vi "TREE_output the selected item.vi"(8 "error in":errorcluster, 10 "only if double click (F)":bool, 11 "Tree In":refnum<vi>) -> (0 "error out":errorcluster, 1 "selected item":string, 2 "selectrd item (path)":path, 3 "Tree Out":refnum<vi>, 4 "directory file names":string[](array[string]))   [LabVIEW 2011]
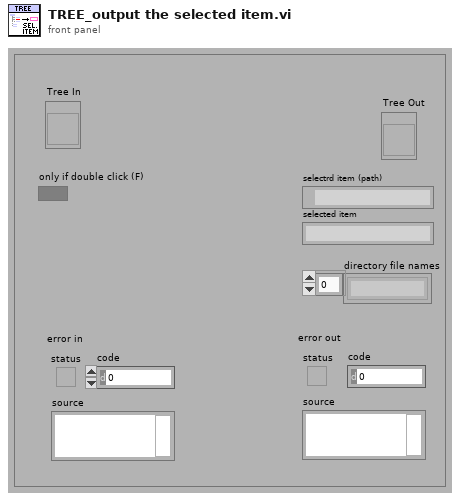
[diagram p1: front panel]
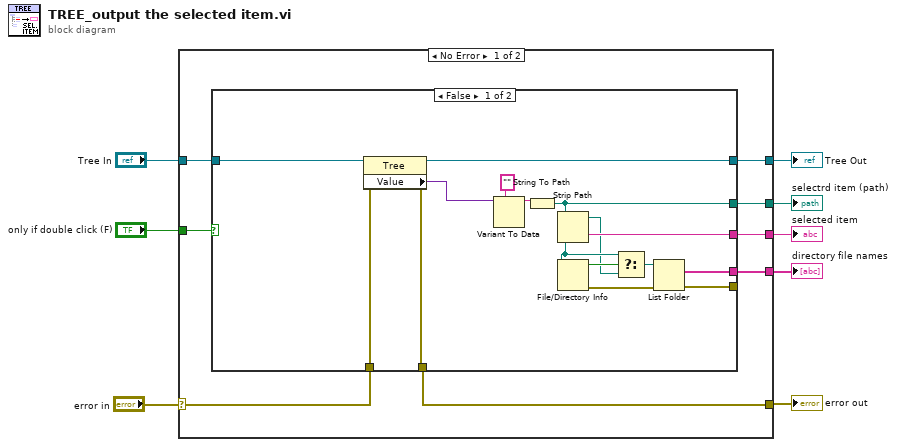
[diagram p0: block diagram]
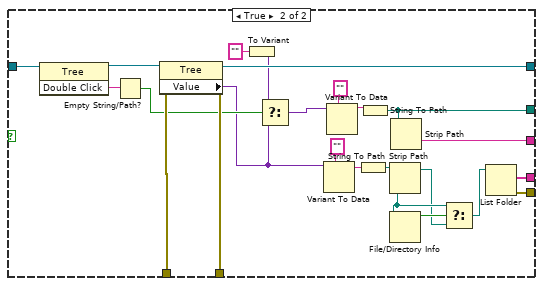
[diagram p2: hidden frame]
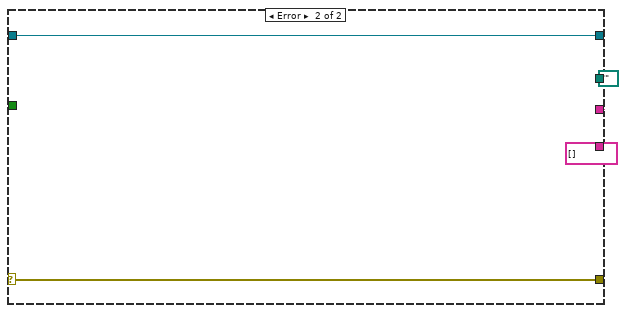
[diagram p3: hidden frame]
diagram:
  n1 = case shown="No Error" "error in" {
    selector: "error in" -> [w15 w58]
    tunnel: "Tree In" -> [w10 w57]
    tunnel: [w10 w57] -> w7
    tunnel: [w9 w58] -> w6
    tunnel: [w14 path ""] -> w4
    tunnel: [w13 "" ("name")] -> w3
    tunnel: "only if double click (F)" -> [w11 _]
    tunnel: [w12 string[] [] ("directory names")] -> w1
    frame No Error {
      n2 = case shown="False" w11 {
        tunnel: [w24 w53] -> _
        tunnel: w15 -> [w29 w52]
        tunnel: [w28 w51] -> w9
        tunnel: [w21 w50] -> w14
        tunnel: w10 -> [w30 w47]
        tunnel: [w23 w42] -> w13
        tunnel: [w19 w33] -> w12
        tunnel: [w16 w31] -> _
        frame False {
          n3 = property class="Tree"(reference=w30, error in=w29) -> (reference out=w24:refnum<vi>, error out=w28:errorcluster, "Value"=w26:variant)
          n4 = Variant To Data(type="", Variant=w26) -> (data=w27:string)  [unwired: 1 in, 1 out]
          n5 = String To Path(string=w27) -> (path=w21:path)
          n6 = Strip Path(path=w21) -> (stripped path=w20:path, name=w23:string)
          n7 = File/Directory Info(path=w21) -> (directory=w22:bool, error out=w18:errorcluster)  [unwired: 1 in, 5 out]
          n8 = Select(t=w21, s=w22, f=w20) -> (s? t:f=w17:path)
          n9 = List Folder(path=w17, error in=w18) -> (filenames=w19:string[], error out=w16:errorcluster)  [unwired: 2 in, 2 out]
        }
        frame True {
          n10 = invoke class="Tree" method="Double Click"(reference=w47) -> (reference out=w48:refnum<vi>, "Double Click"=w49:string)  [unwired: 2 in, 1 out]
          n11 = Empty String/Path?(string/path=w49) -> (empty?=w43:bool)
          n12 = property class="Tree"(reference=w48, error in=w52) -> (reference out=w53:refnum<vi>, error out=w51:errorcluster, "Value"=w37:variant)
          n13 = To Variant(anything="") -> (Variant=w39:variant)
          n14 = Select(t=w39, s=w43, f=w37) -> (s? t:f=w44:variant)
          n15 = Variant To Data(type="", Variant=w37) -> (data=w40:string)  [unwired: 1 in, 1 out]
          n16 = Variant To Data(type="", Variant=w44) -> (data=w45:string)  [unwired: 1 in, 1 out]
          n17 = String To Path(string=w40) -> (path=w35:path)
          n18 = String To Path(string=w45) -> (path=w50:path)
          n19 = Strip Path(path=w35) -> (stripped path=w34:path)  [unwired: 1 out]
          n20 = File/Directory Info(path=w35) -> (directory=w36:bool)  [unwired: 1 in, 6 out]
          n21 = Strip Path(path=w50) -> (name=w42:string)  [unwired: 1 out]
          n22 = Select(t=w35, s=w36, f=w34) -> (s? t:f=w32:path)
          n23 = List Folder(path=w32) -> (filenames=w33:string[], error out=w31:errorcluster)  [unwired: 3 in, 2 out]
        }
      }
    }
    frame Error {
    }
  }
  "Tree Out" <- w7
  "error out" <- w6
  "selectrd item (path)" <- w4
  "selected item" <- w3
  "directory file names" <- w1
